vi "AutoControlsTest.vi"() -> ()   [LabVIEW 2020]
uses:
  <vilib>/Platform/TimedLoop/XDataNode/timing_clust.ctl
  <vilib>/Platform/TimedLoop/XDataNode/nitl_modes.ctl
  <vilib>/Platform/TimedLoop/XDataNode/wakeup.ctl
  <vilib>/platform/TimedLoop/XDataNode/XDataNode.xnode
  <vilib>/Platform/TimedLoop/XDataNode/XDNodeRunTimeDep.lvlib
panel:
  out "current time":timestamp=timestamp(3805970318.2094975 s since 1904-01-01)
  out "PID data out\nIntegrator | In range  | Ki            | Error":dbl[][](array[numeric])=[[1000.0, 1.0, 1.0, 0.0]]
  out "Temperature values":dbl[][](graph)=[[25.0, 25.0]]
  out "Digital control out":cluster{"Inst. #":string, "State":bool}[](array[cluster])=[{"Inst. #"="SSR1", "State"=FALSE}, {"Inst. #"="SSR2", "State"=FALSE}, {"Inst. #"="nan", "State"=FALSE}]
  out "PV1":dbl=nan
  out "Analog values":dbl[][](graph)=[[nan, nan, nan]]
  in  "Setpoints":T1(array[cluster])=[{"Control device"="CD1", "Manual output"=10.0, "Manual | Auto"=FALSE, "Analog | Digital"=FALSE, "Process variable"="PV1", "Setpoint"=30.0, "Control gains"={"Proportional (Kp)"=1.0, "Integral (Ki)"=1.0, "Derivative (Kd)"=0.0}, "Output limits"={"High"=100.0, "Low"=10.0}}]
  out "T02":dbl=25.0
  out "PV3":dbl=nan
  out "T01":dbl=25.0
  out "Analog control out":cluster{"Inst #":string, "Value":dbl}[](array[cluster])=[{"Inst #"="CV1", "Value"=10.0}, {"Inst #"="CV2", "Value"=0.0}, {"Inst #"="CV3", "Value"=0.0}]
  out "PV2":dbl=nan
  in  "stop":bool
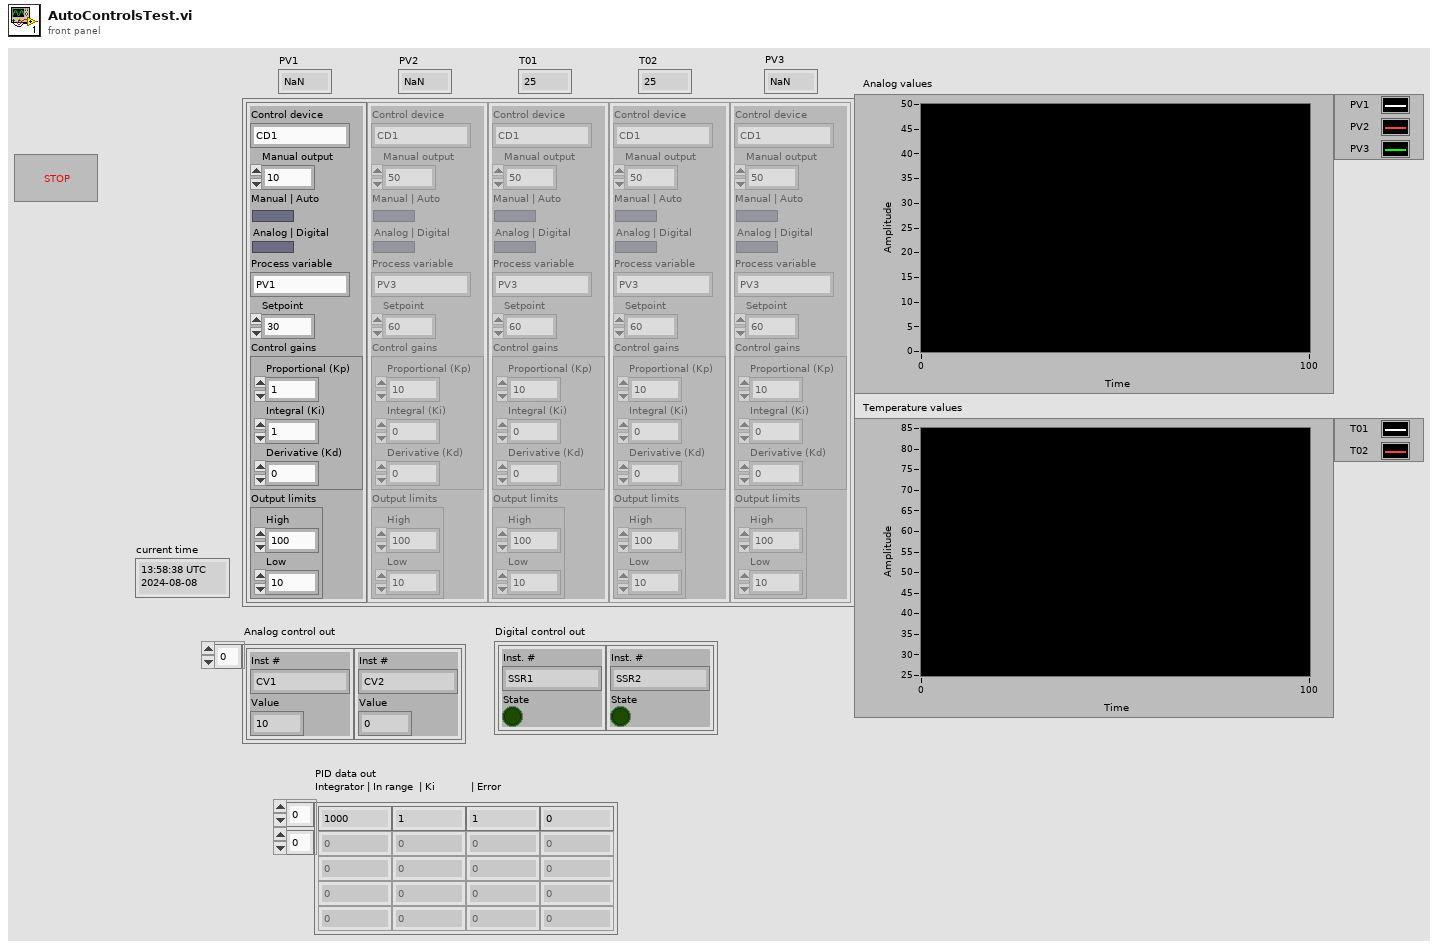
[diagram p1: front panel]
types:
  T1 = cluster{"Control device":string, "Manual output":dbl, "Manual | Auto":bool, "Analog | Digital":bool, "Process variable":string, "Setpoint":dbl, "Control gains":cluster{"Proportional (Kp)":dbl, "Integral (Ki)":dbl, "Derivative (Kd)":dbl}, "Output limits":cluster{"High":dbl, "Low":dbl}}[]
  T2 = typedef "XDNodeRunTimeDep.lvlib/timing_clust.ctl" = cluster{"Expected End [f-1]":u64, "Actual End [f-1]":u64, "Finished Late? [f-1]":bool, "Expected End [i-1]":u64, "Actual End [i-1]":u64, "Finished Late? [i-1]":bool, "Expected Start [i]":u64, "Actual Start [i]":u64, "Expected Start [f]":u64, "Actual Start [f]":u64, "Source Name":string, "Structure Name":string, "Period":i64, "Deadline":i64, "Offset":i64, "Start":i64, "Priority":i32, "Timeout":i32, "Mode":T3, "Wakeup Reason":T4, "Error":errorcluster, "Source Type":string, "Secondary Source Type":string, "Global End Time":u64, "Global Start Time":u64, "Frame Duration":u64, "Iteration Duration":u64, "Assigned CPU":i32, "I/O Scan Engine Mode":u32}
  T3 = typedef "XDNodeRunTimeDep.lvlib/nitl_modes.ctl" = enum32{"No Change", "Process missed periods, maintain original phase", "Discard missed periods, maintain original phase", "Process missed periods, ignore original phase", "Discard missed periods, ignore original phase"}
  T4 = typedef "XDNodeRunTimeDep.lvlib/wakeup.ctl" = enum32{"Normal", "Aborted", "Asynchronous wakeup", "Timing source error", "Timed loop error", "Timeout"}
  T5 = cluster{"Control device":string, "Manual output":dbl, "Manual/Auto":bool, "Analog/Digital":bool, "Process variable":string, "Setpoint":dbl, "Control gains":cluster{"Proportional (Kp)":dbl, "Integral (Ki)":dbl, "Derivative (Kd)":dbl}, "Output limits":cluster{"High":dbl, "Low":dbl}}[]
  T6 = cluster{"Proportional (Kp)":dbl, "Integral (Ki)":dbl, "Derivative (Kd)":dbl}
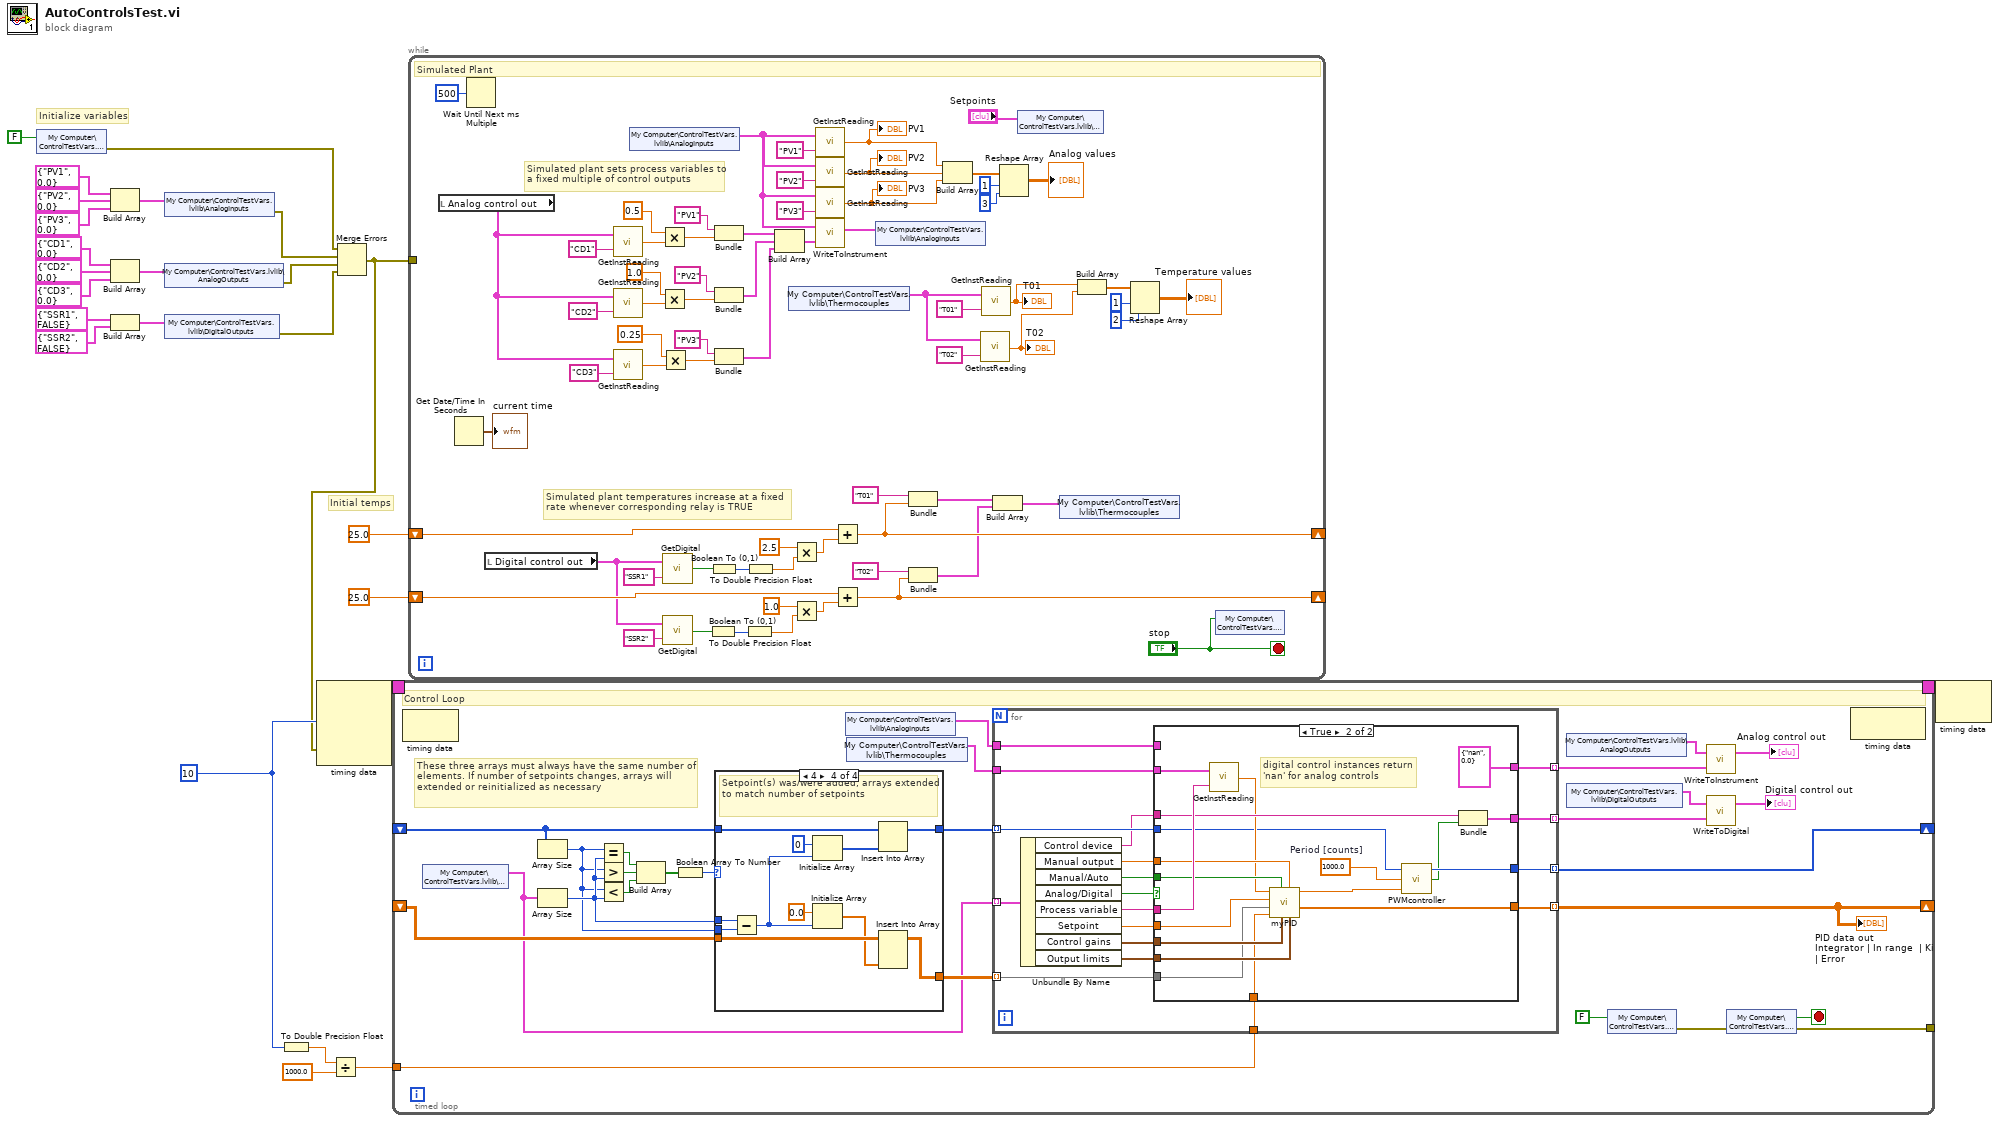
[diagram p0: block diagram]
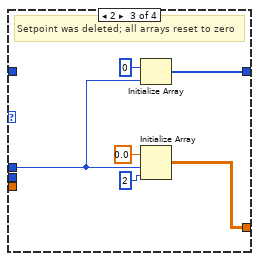
[diagram p4: hidden frame]
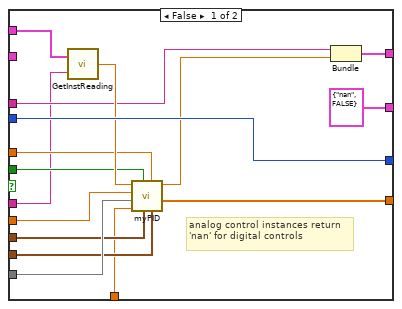
[diagram p5: hidden frame]
diagram:
  w7 = i64 10 ("millisecond multiple")
  # "Initialize variables"
  # "Initial temps"
  n1 = shared-variable "My Computer\\ControlTestVars.lvlib\\STOP"(FALSE ("STOP")) -> (error out=w5:errorcluster)  [unwired: 1 in]
  n2 = Build Array(cluster{string, dbl} {"PV1", 0.0}, cluster{string, dbl} {"PV2", 0.0}, cluster{string, dbl} {"PV3", 0.0}) -> (w22:cluster{string, dbl}[])
  n3 = Build Array(cluster{string, dbl} {"CD1", 0.0}, cluster{string, dbl} {"CD2", 0.0}, cluster{string, dbl} {"CD3", 0.0}) -> (w12:cluster{string, dbl}[])
  n4 = Build Array(cluster{string, bool} {"SSR1", FALSE}, cluster{string, bool} {"SSR2", FALSE}) -> (w16:cluster{string, bool}[])
  n5 = shared-variable "My Computer\\ControlTestVars.lvlib\\AnalogInputs"(w22) -> (error out=w4:errorcluster)  [unwired: 1 in]
  n6 = shared-variable "My Computer\\ControlTestVars.lvlib\\AnalogOutputs"(w12) -> (error out=w3:errorcluster)  [unwired: 1 in]
  n7 = shared-variable "My Computer\\ControlTestVars.lvlib\\DigitalOutputs"(w16) -> (error out=w2:errorcluster)  [unwired: 1 in]
  n8 = To Double Precision Float(number=w7) -> (double precision float=w24:dbl)
  n9 = Divide(x=w24, y=1000.0) -> (x/y=w6:dbl)
  n10 = Merge Errors(w5, w4, w3, w2) -> (w1:errorcluster)
  n11 = node-c288(w7, w1) -> (w9:T2)  [unwired: 2 in]
  n12 = timed-loop {
    tunnel: [w43] -> w20
    shift-right: [w52] -> _
    shift-left: _ -> [w49]
    shift-right: [w29] -> _
    shift-left: _ -> [w48]
    tunnel: w6 -> [w47]
    timing: w9 -> [_]
    timing-out: [_] -> w8
    stop <- w44 stop-if-true
    # "These three arrays must always have the same number of elements. If number of setpoints changes, arrays will extended or reinitialized as necessary"
    # "Control Loop"
    n13 = node-c288() -> ()  [unwired: 1 in, 1 out]
    n14 = shared-variable "My Computer\\ControlTestVars.lvlib\\Setponts"() -> (w28:T5)  [unwired: 1 in, 1 out]
    n15 = Array Size(array=w49) -> (size(s)=w34:i32)
    n16 = Array Size(array=w28) -> (size(s)=w35:i32)
    n17 = Equal?(x=w34, y=w35) -> (x = y?=w40:bool)
    n18 = Greater?(x=w34, y=w35) -> (0:w39:bool)
    n19 = Less?(x=w34, y=w35) -> (x < y?=w38:bool)
    n20 = Build Array(w40, w39, w38) -> (w37:bool[])
    n21 = Boolean Array To Number(Boolean array=w37) -> (number=w36:u32)
    n22 = case shown="4" w36 {
      tunnel: [w56 w58 w63 w74] -> w51
      tunnel: [w55 w57 w60 w68] -> w50
      tunnel: w49 -> [w56 w58 _ w75]
      tunnel: w48 -> [w55 w57 _ w67]
      tunnel: w35 -> [_ _ w62 w73]
      tunnel: w34 -> [_ _ _ w72]
      frame 0, Default {
        # "Default; all arrays passed through"
      }
      frame 1 {
        # "Arrays are equal size and passed through"
      }
      frame 2 {
        # "Setpoint was deleted; all arrays reset to zero"
        n23 = Initialize Array(u32 0 ("element"), w62) -> (w63:u32[])
        n24 = Initialize Array(0.0 ("element"), w62, 2 ("dimension size")) -> (w60:dbl[][])
      }
      frame 4 {
        # "Setpoint(s) was/were added; arrays extended to match number of setpoints"
        n25 = Subtract(x=w73, y=w72) -> (x-y=w70:i32)
        n26 = Initialize Array(u32 0 ("element"), w70) -> (w65:u32[])
        n27 = Initialize Array(0.0 ("element"), w70) -> (w66:dbl[])
        n28 = Insert Into Array(array=w75, new element=w65) -> (w74:u32[])  [unwired: 1 in]
        n29 = Insert Into Array(array=w67, new element=w66) -> (w68:dbl[][])  [unwired: 2 in]
      }
    }
    n30 = shared-variable "My Computer\\ControlTestVars.lvlib\\AnalogInputs"() -> (w46:cluster{"Inst. #":string, "Value":dbl}[])  [unwired: 1 in, 1 out]
    n31 = shared-variable "My Computer\\ControlTestVars.lvlib\\Thermocouples"() -> (w45:cluster{"Inst. #":string, "Value":dbl}[])  [unwired: 1 in, 1 out]
    n32 = for {
      tunnel: [w93] -> w52 mode=indexing
      tunnel: w51 -> [w92] mode=indexing
      tunnel: w45 -> [w91]
      tunnel: [w90] -> w30 mode=indexing
      tunnel: [w89] -> w32 mode=indexing
      tunnel: w28 -> [w76] mode=indexing
      tunnel: [w88] -> w29 mode=indexing
      tunnel: w50 -> [w87] mode=indexing
      tunnel: w46 -> [w78]
      tunnel: w47 -> [w77]
      n33 = Unbundle By Name(w76) -> ("Control device"=w86:string, "Manual output"=w85:dbl, "Manual/Auto"=w84:bool, "Analog/Digital"=w83:bool, "Process variable"=w82:string, "Setpoint"=w81:dbl, "Control gains"=w80:T6, "Output limits"=w79:cluster{"High":dbl, "Low":dbl})
      n34 = case shown="True" w83 {
        tunnel: [w97 cluster{string, "Period [ms]":dbl} {"nan", "Period [ms]"=0.0}] -> w90
        tunnel: [w108 w113] -> w93
        tunnel: w92 -> [w108 w114]
        tunnel: w91 -> [_ w128]
        tunnel: [cluster{string, bool} {"nan", FALSE} w124] -> w89
        tunnel: [w107 w116] -> w88
        tunnel: w87 -> [w106 w115]
        tunnel: w86 -> [w104 w125]
        tunnel: w85 -> [w103 w120]
        tunnel: w84 -> [w102 w121]
        tunnel: w82 -> [w101 w126]
        tunnel: w81 -> [w100 w118]
        tunnel: w80 -> [w99 w123]
        tunnel: w79 -> [w98 w122]
        tunnel: w78 -> [w96 _]
        tunnel: w77 -> [w95 w119]
        frame False {
          # "analog control instances return 'nan' for digital controls"
          n35 = call "GetInstReading.vi"("Inst number"=w101, "Array"=w96) -> ("Reading"=w105:dbl)
          n36 = call "myPID.vi"("Output limits"=w98, "manual input"=w103, "PID gains"=w99, "manual/auto"=w102, "dt (s)"=w95, "PID data in"=w106, "setpoint"=w100, "process variable"=w105) -> ("PID data out"=w107:dbl[], "Output"=w94:dbl)  [unwired: 2 in]
          n37 = Bundle("Control device"=w104, "Output"=w94) -> (w97:cluster{"Control device":string, "Output":dbl})  [unwired: 1 in]
        }
        frame True {
          w111 = 1000.0  # Period [counts]
          # "digital control instances return\n'nan' for analog controls"
          n38 = call "GetInstReading.vi"("Inst number"=w126, "Array"=w128) -> ("Reading"=w117:dbl)
          n39 = call "myPID.vi"("Output limits"=w122, "manual input"=w120, "PID gains"=w123, "manual/auto"=w121, "dt (s)"=w119, "PID data in"=w115, "setpoint"=w118, "process variable"=w117) -> ("PID data out"=w116:dbl[], "Output"=w110:dbl)  [unwired: 2 in]
          n40 = call "PWMcontroller.vi"("Duty Cycle [0-100%]"=w110, "Period [ms]"=w111, "Count in"=w114) -> ("State"=w112:bool, "Count out"=w113:u32)  [unwired: 1 in]
          n41 = Bundle("Control device"=w125, "State"=w112) -> (w124:cluster{"Control device":string, "State":bool})  [unwired: 1 in]
        }
      }
    }
    "PID data out\nIntegrator | In range  | Ki            | Error" <- w29
    n42 = shared-variable "My Computer\\ControlTestVars.lvlib\\AnalogOutputs"() -> (w42:cluster{"Inst. #":string, "Value":dbl}[])  [unwired: 1 in, 1 out]
    n43 = shared-variable "My Computer\\ControlTestVars.lvlib\\DigitalOutputs"() -> (w33:cluster{"Inst. #":string, "State":bool}[])  [unwired: 1 in, 1 out]
    n44 = call "WriteToInstrument.vi"("New values"=w30, "Inst. array in"=w42) -> ("Inst. array out"=→"Analog control out":cluster{"Inst #":string, "Value":dbl}[])  [unwired: 1 in]
    n45 = call "WriteToDigital.vi"("New DO"=w32, "DO in"=w33) -> ("DO out"=→"Digital control out":cluster{"Inst. #":string, "State":bool}[])  [unwired: 1 in]
    n46 = shared-variable "My Computer\\ControlTestVars.lvlib\\STOP"() -> (w44:bool, error out=w43:errorcluster)  [unwired: 1 in]
    n47 = node-c288() -> ()  [unwired: 1 in, 1 out]
  }
  n48 = while {
    shift-right: [w180] -> _
    shift-left: 25.0 -> [w181]
    shift-right: [w163] -> _
    shift-left: 25.0 -> [w173]
    tunnel: w1 -> [_]
    stop <- "stop" stop-if-true
    # "Simulated plant sets process variables to a fixed multiple of control outputs"
    # "Simulated plant temperatures increase at a fixed rate whenever corresponding relay is TRUE"
    # "Simulated Plant"
    n49 = local read "Analog control out"() -> (w142:cluster{"Inst #":string, "Value":dbl}[])
    n50 = Get Date/Time In Seconds() -> (seconds since 1Jan1904=→"current time":timestamp)
    n51 = Wait Until Next ms Multiple(millisecond multiple=u32 500) -> ()  [unwired: 1 out]
    n52 = local read "Digital control out"() -> (w140:cluster{"Inst. #":string, "State":bool}[])
    n53 = call "GetInstReading.vi"("Inst number"="CD1", "Array"=w142) -> ("Reading"=w147:dbl)
    n54 = call "GetInstReading.vi"("Inst number"="CD2", "Array"=w142) -> ("Reading"=w156:dbl)
    n55 = call "GetInstReading.vi"("Inst number"="CD3", "Array"=w142) -> ("Reading"=w146:dbl)
    n56 = shared-variable "My Computer\\ControlTestVars.lvlib\\AnalogInputs"() -> (w153:cluster{"Inst. #":string, "Value":dbl}[])  [unwired: 1 in, 1 out]
    n57 = Multiply(x=0.5, y=w147) -> (x*y=w188:dbl)
    n58 = Multiply(x=1.0, y=w156) -> (x*y=w141:dbl)
    n59 = Multiply(x=0.25, y=w146) -> (x*y=w152:dbl)
    n60 = call "GetDigital.vi"("Inst number"="SSR1", "Array"=w140) -> ("State"=w186:bool)
    n61 = call "GetDigital.vi"("Inst number"="SSR2", "Array"=w140) -> ("State"=w174:bool)
    n62 = Boolean To (0,1)(Boolean=w174) -> (0, 1=w176:i16)
    n63 = Boolean To (0,1)(Boolean=w186) -> (0, 1=w184:i16)
    n64 = Bundle("PV1", w188) -> (w193:cluster{string, dbl})  [unwired: 1 in]
    n65 = Bundle("PV2", w141) -> (w164:cluster{string, dbl})  [unwired: 1 in]
    n66 = Bundle("PV3", w152) -> (w148:cluster{string, dbl})  [unwired: 1 in]
    n67 = To Double Precision Float(number=w176) -> (double precision float=w177:dbl)
    n68 = To Double Precision Float(number=w184) -> (double precision float=w183:dbl)
    n69 = Build Array(w193, w164, w148) -> (w158:cluster{string, dbl}[])
    n70 = shared-variable "My Computer\\ControlTestVars.lvlib\\Thermocouples"() -> (w161:cluster{"Inst. #":string, "Value":dbl}[])  [unwired: 1 in, 1 out]
    n71 = Multiply(x=2.5, y=w183) -> (x*y=w182:dbl)
    n72 = Multiply(x=1.0, y=w177) -> (x*y=w171:dbl)
    n73 = call "GetInstReading.vi"("Inst number"="PV1", "Array"=w153) -> ("Reading"=w139:dbl)
    "PV1" <- w139
    n74 = call "GetInstReading.vi"("Inst number"="PV2", "Array"=w153) -> ("Reading"=w138:dbl)
    "PV2" <- w138
    n75 = call "GetInstReading.vi"("Inst number"="PV3", "Array"=w153) -> ("Reading"=w137:dbl)
    "PV3" <- w137
    n76 = call "WriteToInstrument.vi"("New values"=w158, "Inst. array in"=w153) -> ("Inst. array out"=w157:cluster{"Inst #":string, "Value":dbl}[])  [unwired: 1 in]
    n77 = Add(x=w181, y=w182) -> (x+y=w180:dbl)
    n78 = Add(x=w173, y=w171) -> (x+y=w163:dbl)
    n79 = shared-variable "My Computer\\ControlTestVars.lvlib\\AnalogInputs"(w157) -> ()  [unwired: 1 in, 1 out]
    n80 = Bundle("T01", w180) -> (w191:cluster{string, dbl})  [unwired: 1 in]
    n81 = Bundle("T02", w163) -> (w170:cluster{string, dbl})  [unwired: 1 in]
    n82 = Build Array(w139, w138, w137) -> (w145:dbl[])
    n83 = call "GetInstReading.vi"("Inst number"="T02", "Array"=w161) -> ("Reading"=w134:dbl)
    "T02" <- w134
    n84 = call "GetInstReading.vi"("Inst number"="T01", "Array"=w161) -> ("Reading"=w135:dbl)
    "T01" <- w135
    n85 = Build Array(w191, w170) -> (w160:cluster{string, dbl}[])
    n86 = Reshape Array(w145, 1 ("dimension size"), 3 ("dimension size")) -> (→"Analog values":dbl[][])
    n87 = shared-variable "My Computer\\ControlTestVars.lvlib\\Setponts"("Setpoints") -> ()  [unwired: 1 in, 1 out]
    n88 = shared-variable "My Computer\\ControlTestVars.lvlib\\Thermocouples"(w160) -> ()  [unwired: 1 in, 1 out]
    n89 = Build Array(w135, w134) -> (w133:dbl[])
    n90 = Reshape Array(w133, 1 ("dimension size"), 2 ("dimension size")) -> (→"Temperature values":dbl[][])
    n91 = shared-variable "My Computer\\ControlTestVars.lvlib\\STOP"("stop") -> ()  [unwired: 1 in, 1 out]
  }
  n92 = shared-variable "My Computer\\ControlTestVars.lvlib\\STOP"(FALSE ("STOP"), error in=w20) -> ()  [unwired: 1 out]
  n93 = node-c288(w8) -> ()  [unwired: 1 out]
